vi "PH_Sequencer.ProcEvents.vi"(0 "i ref in":refnum<vi>, 5 "error in (no error)":errorcluster) -> (14 "i ref out":refnum<vi>, 19 "error out":errorcluster)   [LabVIEW 2014, in "PH_Sequencer.lvlib"]
doc: "This method is used to define the events the object will listen to. Add your own events here."
uses:
  PH_Sequencer.lvlib
  CS_Core/BaseProcess/BaseProcess.event definition.ctl
  CS_Core/CAEObj/CAEObj.event definition.ctl
  CS_Core/BaseProcess/BaseProcess.descriptor string definition.ctl
  PH_Basics/PH_PowerUnit_BaseClass/PH_PowerUnit_BaseClass.PP PU Tags.ctl
  PH_Basics/PH_PP_Common/PH_PP_Common.PUs.ctl
  PH_Devices/PH_Beckhoff_PP_PU/PH_Beckhoff_PP_PU.HV Meas Tags.ctl
  CS_Core/BaseProcess/BaseProcess.lvlib
  CS_Core/CAEObj/CAEObj.lvlib
  PH_Basics/PH_Common/PH_Common.lvlib
  PH_Devices/PH_Beckhoff_PP_PU/PH_Beckhoff_PP_PU.lvlib
  PH_Basics/PH_PowerUnit_BaseClass/PH_PowerUnit_BaseClass.lvlib
  PH_Basics/PH_PP_Common/PH_PP_Common.lvlib
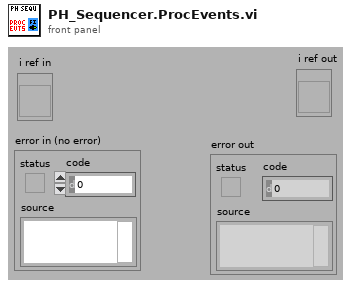
[diagram p1: front panel]
types:
  T1 = typedef "PH_PP_Common.lvlib/PH_PP_Common.PUs.ctl" = enum16{"no Info", "PA-19mm-1", "PA-19mm-2", "PA-45mm-PILC", "PA-45mm-MAIN", "MA-PU-1", "MA-PU-2", "MA-PU-3", "MA-PU-4", "MA-PU-5", "MA-PU-6", "MA-FR", "MA-PILC", "PA-45mm-DP"}
  T2 = typedef "PH_PowerUnit_BaseClass.lvlib/PH_PowerUnit_BaseClass.PP PU Tags.ctl" = enum16{"Waiting-Time", "PU-in-Use"}
  T3 = typedef "BaseProcess.lvlib/BaseProcess.event definition.ctl" = cluster{"CAEEvtDef":T4, "Data Descriptor":T5}
  T4 = typedef "CAEObj.lvlib/CAEObj.event definition.ctl" = cluster{"URL":string, "enable":bool, "ignoreResID":bool}
  T5 = typedef "BaseProcess.lvlib/BaseProcess.descriptor string definition.ctl" = string
  T6 = typedef "PH_Beckhoff_PP_PU.lvlib/PH_Beckhoff_PP_PU.HV Meas Tags.ctl" = enum16{"voltage-raw", "voltage"}
  T7 = typedef "PH_Sequencer.lvlib/PH_Sequencer.i attribute.ctl" = cluster{"GUI Refs":cluster{"Main Off":refnum<vi>, "Fire":refnum<vi>, "Status":refnum<vi>, "Ready":refnum<vi>, "Waiting Time":refnum<vi>, "Timeout":refnum<vi>, "PPMA Ready":refnum<vi>, "Sequencer SM State":refnum<vi>, "PPPA Ready":refnum<vi>, "Calorimeter":refnum<vi>, "Beamline Ready":refnum<vi>, "Clear Beamline":refnum<vi>, "Linkage PPMA Rods":refnum<vi>, "Linkage Current PA":refnum<vi>, "Linkage Current MA":refnum<vi>, "Timing Ready":refnum<vi>, "State Timing":refnum<vi>, "Force Timing":refnum<vi>, "PSDB Shot Comment":refnum<vi>, "State PA Backreflection":refnum<vi>, "Beamline Z6 Ready":refnum<vi>, "Clear Z6 Beamline":refnum<vi>, "Sequence length":refnum<vi>, "Timing Mode":refnum<vi>, "Slow Trigger Settings":refnum<vi>, "Experiment Description":refnum<vi>, "State PSDB":refnum<vi>, "PSDB Ready":refnum<vi>, "Set PSDB Settings":refnum<vi>, "Get PSDB Info":refnum<vi>, "Take Snapshot":refnum<vi>, "Shottype":refnum<vi>, "Experiment":refnum<vi>, "Phase Frontends":refnum<vi>, "PP 45mm PILC in use":refnum<vi>}, "Status Info":cluster{"Machine Status":T8, "WaitingTime":i32, "Timeout":bool}, "Readyness":cluster{"Ready to shot":bool, "PPMA Ready":bool, "PPPA Ready":bool, "BL Ready":bool, "Timing Ready":bool, "BL Z6 Ready":bool, "PSDBReady":bool}, "Instancenames":cluster{"PPMA Rods":string, "PP Current Meas":string, "PH Beamline Chief":string, "PA Backrefl Meas":string, "Z6 Beamline Chief":string}, "Data to read":bool, "Calorimeter":cluster{"Instancename":string, "On":bool, "linked":bool}, "Linkage":cluster{"PPMA Rods":bool, "PP Current Meas":bool, "PHELIX Beamline Chief":bool, "PA Backrefl Meas":bool, "Z6 Beamline Chief":bool}, "Timing":cluster{"Instance":string, "linked":bool, "Status":T8, "Timing Mode":T9, "Slow Trigger Settings":T10, "Info available":cluster{"ext SlowTrigger":bool, "T2":bool, "Mode":bool, "Delay Slow Trigger":bool, "Phase FEs":bool}, "FE Phase":T11}, "Service ID R2S":i32, "PSDB":cluster{"Controller Instance":string, "Controller Status":T8, "Controller linked":bool, "Settings acknowledged":bool, "Current Experiment ID":i16, "Current Shot Type":i16, "Current Comment":string, "Remember Settings":bool, "Write 2 early":bool}, "PSDB Data":cluster{"Main Off?":bool, "Sequence Length":dbl, "Sequence startet":timestamp}, "6P 4Q Positions":cluster{"Instancename":string, "linked":bool, "Position":T12}[], "PUs":T13[]}
  T8 = typedef "PH_StatusHandler.lvlib/PH_StatusHandler.Status.ctl" = i16
  T9 = typedef "PH_Timing.lvlib/PH_Timing.Timing Mode.ctl" = cluster{"T2":i16, "Modeselector":enum32{"10 Hz", "0.5 Hz", "Shot"}}
  T10 = typedef "PH_Timing.lvlib/PH_Timing.Slow Trigger Settings.ctl" = cluster{"Delay":dbl, "externally triggered?":bool}
  T11 = typedef "PH_Timing.lvlib/PH_Timing.Phase FEs.ctl" = cluster{"Phase":dbl}
  T12 = typedef "PH_4_Pos_Selector.lvlib/PH_4_Pos_Selector.Position Selector.ctl" = u16
  T13 = typedef "PH_Sequencer.lvlib/PH_Sequencer.Head.ctl" = cluster{"PowerUnit":T1, "GUI Ref":refnum<vi>, "Information":T14, "linked?":bool, "GUI Ref Current Voltage":refnum<vi>}
  T14 = typedef "PH_Sequencer.lvlib/PH_Sequencer.PU Information.ctl" = cluster{"State":T8, "Waiting Time [s]":dbl, "PU State SM":T15, "PU Timeout SM":T15}
  T15 = typedef "PH_PowerUnit_BaseClass.lvlib/PH_PowerUnit_BaseClass.SM States.ctl" = enum16{".", "Stand by", "Switch PU on", "Configure", "Set Default Voltage", "Set STANDBY", "Set READY", "Wait for Shot Cmd", "Open Dump Rods", "Open Ross Relais", "Close Ross Relais", "Switch PSU on", "Switch PSU off", "Charge", "Switch GD Channel on", "Close Dump Rods", "Rods-TO", "RR-TO", "PSU-TO", "Trigger-TO"}
  T16 = cluster{"Instancename":string, "linked":bool, "Position":T12}[]
  T17 = typedef "PH_Common.lvlib/PH_DIM.Event Declarer.ctl" = cluster{"Service Name":string, "Selector":string}
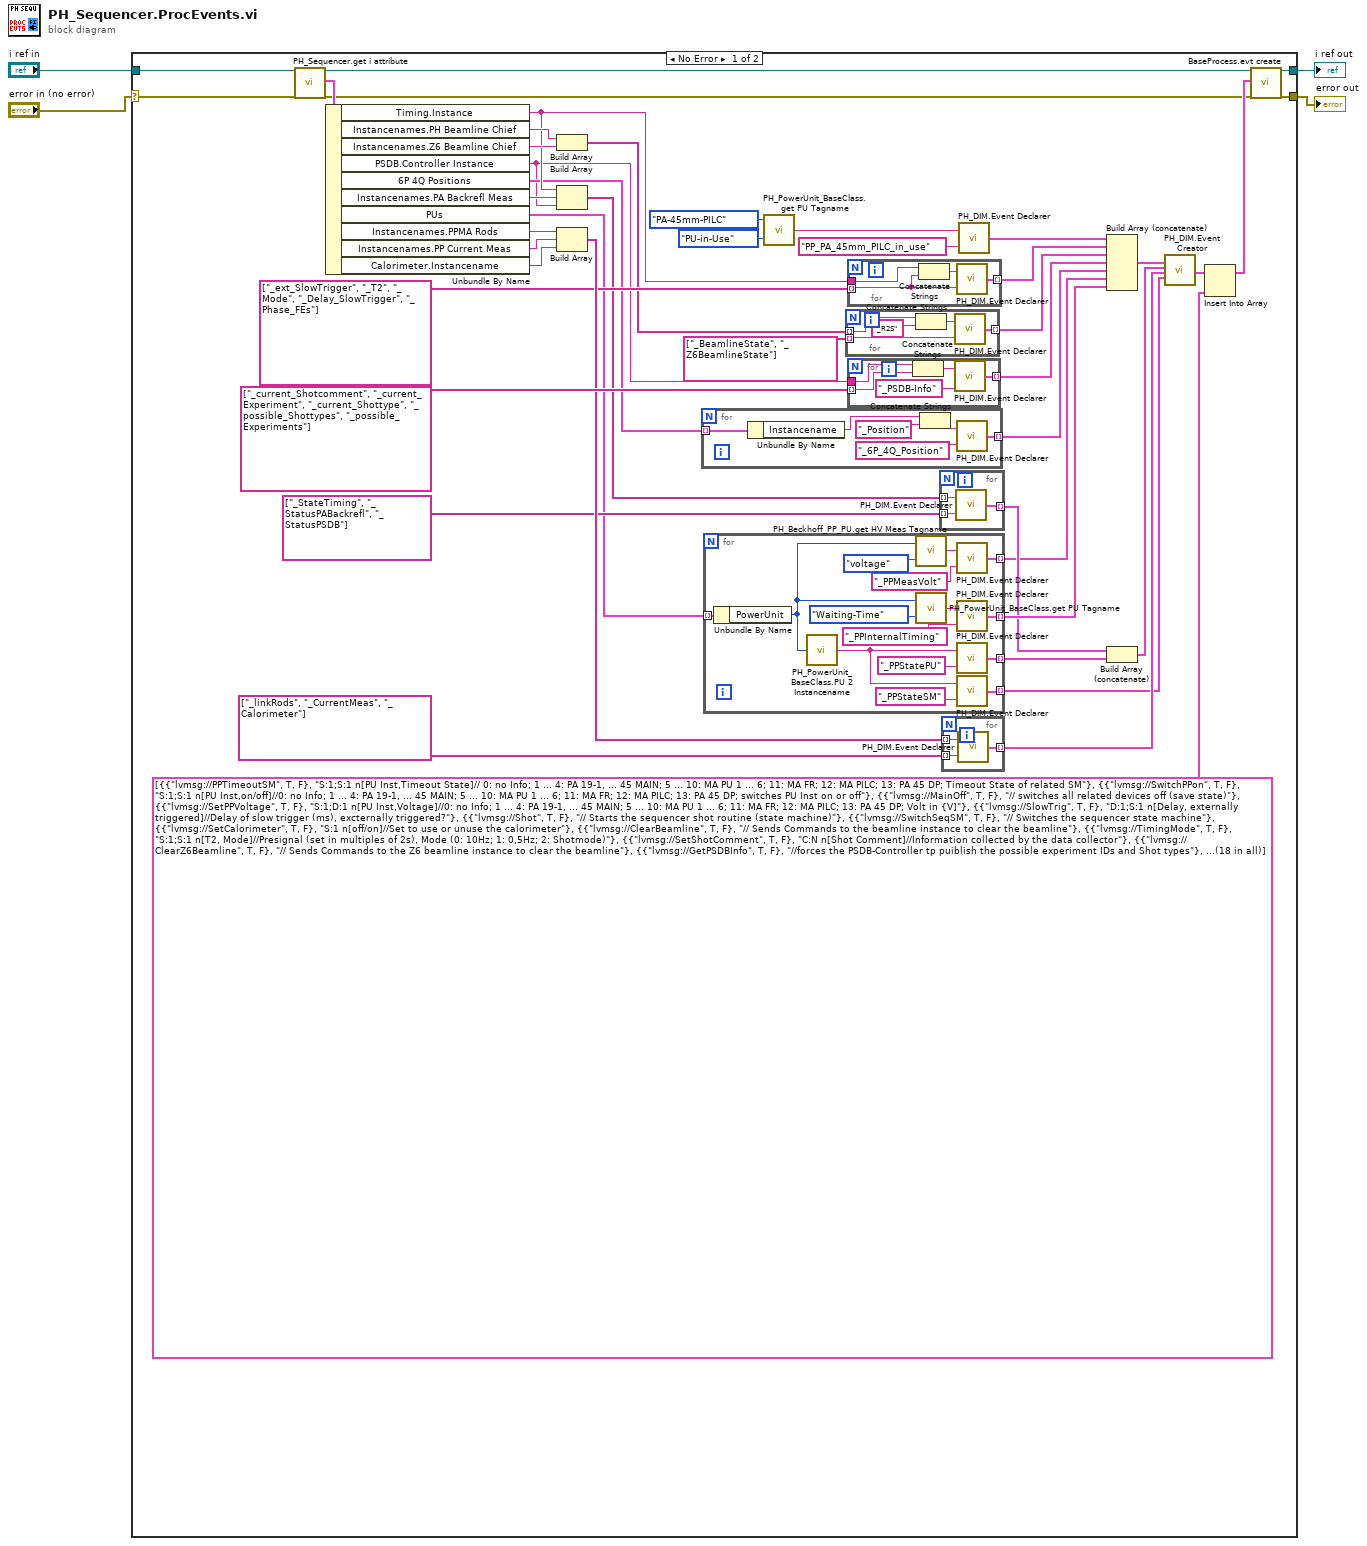
[diagram p0: block diagram]
diagram:
  n1 = case shown="No Error" "error in (no error)" {
    selector: "error in (no error)" -> [w44 w91]
    tunnel: "i ref in" -> [w47 w92]
    tunnel: [w46 w92] -> w3
    tunnel: [w45 w91] -> w2
    frame No Error {
      n2 = call "PH_Sequencer.get i attribute.vi"("i ref in"=w47, "error in (no error)"=w44) -> ("i ref out"=w49:refnum<vi>, "i attribute"=w32:T7, "error out"=w6:errorcluster)  [unwired: 15 in]
      n3 = Unbundle By Name(w32) -> ("Timing.Instance"=w21:string, "Instancenames.PH Beamline Chief"=w29:string, "Instancenames.Z6 Beamline Chief"=w28:string, "PSDB.Controller Instance"=w14:string, "6P 4Q Positions"=w18:T16, "Instancenames.PA Backrefl Meas"=w26:string, "PUs"=w16:T13[], "Instancenames.PPMA Rods"=w25:string, "Instancenames.PP Current Meas"=w24:string, "Calorimeter.Instancename"=w23:string)
      n4 = Build Array(w29, w28) -> (w13:string[])
      n5 = Build Array(w21, w26, w14) -> (w22:string[])
      n6 = Build Array(w25, w24, w23) -> (w38:string[])
      n7 = for {
        tunnel: [w53] -> w17 mode=indexing
        tunnel: w18 -> [w51] mode=indexing
        n8 = Unbundle By Name(w51) -> ("Instancename"=w50:string)
        n9 = Concatenate Strings(w50, "_Position" ("string")) -> (w55:string)
        n10 = call "PH_DIM.Event Declarer.vi"("Selector"="_6P_4Q_Position", "Service Name"=w55) -> ("declared DIM Event"=w53:T17)
      }
      n11 = for {
        tunnel: [w89] -> w39 mode=indexing
        tunnel: [w88] -> w34 mode=indexing
        tunnel: w16 -> [w86] mode=indexing
        tunnel: [w84] -> w9 mode=indexing
        tunnel: [w77] -> w8 mode=indexing
        n12 = Unbundle By Name(w86) -> ("PowerUnit"=w78:T1)
        n13 = call "PH_PowerUnit_BaseClass.PU 2 Instancename.vi"("PU"=w78) -> ("Instance Name"=w85:string)
        n14 = call "PH_Beckhoff_PP_PU.get HV Meas Tagname.vi"("HV Meas Tag"=PH_Beckhoff_PP_PU.HV_Meas_Tags."voltage", "PU"=w78) -> ("HV Meas Tagname"=w80:string)
        n15 = call "PH_PowerUnit_BaseClass.get PU Tagname.vi"("PU Tag"=PH_PowerUnit_BaseClass.PP_PU_Tags."Waiting-Time", "PU"=w78) -> ("PU Tagname"=w82:string)
        n16 = call "PH_DIM.Event Declarer.vi"("Selector"="_PPMeasVolt" ("URL"), "Service Name"=w80) -> ("declared DIM Event"=w77:T17)
        n17 = call "PH_DIM.Event Declarer.vi"("Selector"="_PPInternalTiming" ("URL"), "Service Name"=w82) -> ("declared DIM Event"=w89:T17)
        n18 = call "PH_DIM.Event Declarer.vi"("Selector"="_PPStatePU" ("URL"), "Service Name"=w85) -> ("declared DIM Event"=w88:T17)
        n19 = call "PH_DIM.Event Declarer.vi"("Selector"="_PPStateSM" ("URL"), "Service Name"=w85) -> ("declared DIM Event"=w84:T17)
      }
      n20 = call "PH_PowerUnit_BaseClass.get PU Tagname.vi"("PU Tag"=PH_PowerUnit_BaseClass.PP_PU_Tags."PU-in-Use", "PU"=PH_PP_Common.PUs."PA-45mm-PILC") -> ("PU Tagname"=w11:string)
      n21 = for {
        tunnel: [w75] -> w40 mode=indexing
        tunnel: w13 -> [w73] mode=indexing
        tunnel: string[] ["_BeamlineState", "_Z6BeamlineState"] -> [w74] mode=indexing
        n22 = Concatenate Strings(w73, "_R2S" ("string")) -> (w72:string)
        n23 = call "PH_DIM.Event Declarer.vi"("Selector"=w74, "Service Name"=w72) -> ("declared DIM Event"=w75:T17)
      }
      n24 = for {
        tunnel: [w59] -> w27 mode=indexing
        tunnel: w21 -> [w57]
        tunnel: string[] ["_ext_SlowTrigger", "_T2", "_Mode", "_Delay_SlowTrigger", "_Phase_FEs"] -> [w56] mode=indexing
        n25 = Concatenate Strings(w57, w56) -> (w58:string)
        n26 = call "PH_DIM.Event Declarer.vi"("Selector"=w56, "Service Name"=w58) -> ("declared DIM Event"=w59:T17)
      }
      n27 = for {
        tunnel: w14 -> [w64]
        tunnel: string[] ["_current_Shotcomment", "_current_Experiment", "_current_Shottype", "_possible_Shottypes", "_possible_Experiments"] -> [w63] mode=indexing
        tunnel: [w60] -> w41 mode=indexing
        n28 = Concatenate Strings(w64, w63) -> (w62:string)
        n29 = call "PH_DIM.Event Declarer.vi"("Selector"="_PSDB-Info" ("URL"), "Service Name"=w62) -> ("declared DIM Event"=w60:T17)
      }
      n30 = for {
        tunnel: [w65] -> w35 mode=indexing
        tunnel: w22 -> [w67] mode=indexing
        tunnel: string[] ["_StateTiming", "_StatusPABackrefl", "_StatusPSDB"] -> [w66] mode=indexing
        n31 = call "PH_DIM.Event Declarer.vi"("Selector"=w66, "Service Name"=w67) -> ("declared DIM Event"=w65:T17)
      }
      n32 = for {
        tunnel: [w68] -> w15 mode=indexing
        tunnel: w38 -> [w69] mode=indexing
        tunnel: string[] ["_linkRods", "_CurrentMeas", "_Calorimeter"] -> [w70] mode=indexing
        n33 = call "PH_DIM.Event Declarer.vi"("Selector"=w70, "Service Name"=w69) -> ("declared DIM Event"=w68:T17)
      }
      n34 = call "PH_DIM.Event Declarer.vi"("Selector"="PP_PA_45mm_PILC_in_use", "Service Name"=w11) -> ("declared DIM Event"=w7:T17)
      n35 = Build Array (concatenate)(w7, w27, w40, w41, w17, w8, w39) -> (w42:T17[])
      n36 = Build Array (concatenate)(w35, w34) -> (w36:T17[])
      n37 = call "PH_DIM.Event Creator.vi"("Trendmessage Services"=w42, "Status Services"=w36, "condition Services"=w15, "SM State Services"=w9) -> ("DIM Service Events"=w20:T3[])  [unwired: 15 in]
      n38 = Insert Into Array(array=w20, new element=T3[] [{"CAEEvtDef"={"URL"="lvmsg://PPTimeoutSM", "enable"=TRUE, "ignoreResID"=FALSE}, "Data Descriptor"="S:1;S:1 n[PU Inst,Timeout State]// 0: no Info; 1 ... 4: PA 19-1, ... 45 MAIN; 5 ... 10: MA PU 1 ... 6; 11: MA FR; 12: MA PILC; 13: PA 45 DP; Timeout State of related SM"}, {"CAEEvtDef"={"URL"="lvmsg://SwitchPPon", "enable"=TRUE, "ignoreResID"=FALSE}, "Data Descriptor"="S:1;S:1 n[PU Inst,on/off]//0: no Info; 1 ... 4: PA 19-1, ... 45 MAIN; 5 ... 10: MA PU 1 ... 6; 11: MA FR; 12: MA PILC; 13: PA 45 DP; switches PU Inst on or off"}, {"CAEEvtDef"={"URL"="lvmsg://MainOff", "enable"=TRUE, "ignoreResID"=FALSE}, "Data Descriptor"="// switches all related devices off (save state)"}, {"CAEEvtDef"={"URL"="lvmsg://SetPPVoltage", "enable"=TRUE, "ignoreResID"=FALSE}, "Data Descriptor"="S:1;D:1 n[PU Inst,Voltage]//0: no Info; 1 ... 4: PA 19-1, ... 45 MAIN; 5 ... 10: MA PU 1 ... 6; 11: MA FR; 12: MA PILC; 13: PA 45 DP; Volt in {V]"}, {"CAEEvtDef"={"URL"="lvmsg://SlowTrig", "enable"=TRUE, "ignoreResID"=FALSE}, "Data Descriptor"="D:1;S:1 n[Delay, externally triggered]//Delay of slow trigger (ms), excternally triggered?"}, {"CAEEvtDef"={"URL"="lvmsg://Shot", "enable"=TRUE, "ignoreResID"=FALSE}, "Data Descriptor"="// Starts the sequencer shot routine (state machine)"}, {"CAEEvtDef"={"URL"="lvmsg://SwitchSeqSM", "enable"=TRUE, "ignoreResID"=FALSE}, "Data Descriptor"="// Switches the sequencer state machine"}, {"CAEEvtDef"={"URL"="lvmsg://SetCalorimeter", "enable"=TRUE, "ignoreResID"=FALSE}, "Data Descriptor"="S:1 n[off/on]//Set to use or unuse the calorimeter"}, {"CAEEvtDef"={"URL"="lvmsg://ClearBeamline", "enable"=TRUE, "ignoreResID"=FALSE}, "Data Descriptor"="// Sends Commands to the beamline instance to clear the beamline"}, {"CAEEvtDef"={"URL"="lvmsg://TimingMode", "enable"=TRUE, "ignoreResID"=FALSE}, "Data Descriptor"="S:1;S:1 n[T2, Mode]//Presignal (set in multiples of 2s), Mode (0: 10Hz; 1: 0,5Hz; 2: Shotmode)"}, {"CAEEvtDef"={"URL"="lvmsg://SetShotComment", "enable"=TRUE, "ignoreResID"=FALSE}, "Data Descriptor"="C:N n[Shot Comment]//Information collected by the data collector"}, {"CAEEvtDef"={"URL"="lvmsg://ClearZ6Beamline", "enable"=TRUE, "ignoreResID"=FALSE}, "Data Descriptor"="// Sends Commands to the Z6 beamline instance to clear the beamline"}, {"CAEEvtDef"={"URL"="lvmsg://GetPSDBInfo", "enable"=TRUE, "ignoreResID"=FALSE}, "Data Descriptor"="//forces the PSDB-Controller tp puiblish the possible experiment IDs and Shot types"}, {"CAEEvtDef"={"URL"="lvmsg://SetExpID", "enable"=TRUE, "ignoreResID"=FALSE}, "Data Descriptor"="S:1 n[Experiment ID]//sends the wanted Experiment ID to the PSDB-Controller"}, {"CAEEvtDef"={"URL"="lvmsg://SetShotType", "enable"=TRUE, "ignoreResID"=FALSE}, "Data Descriptor"="S:1 n[Shot Type]//sends the wanted Shot Type to the PSDB-Controller"}, {"CAEEvtDef"={"URL"="lvmsg://SetPSDBSettings", "enable"=TRUE, "ignoreResID"=FALSE}, "Data Descriptor"="// confirms by setting own attributes that PSDB-Settings are checked"}, {"CAEEvtDef"={"URL"="lvmsg://GetPSDBSnapshot", "enable"=TRUE, "ignoreResID"=FALSE}, "Data Descriptor"="// requests a PSDB Snapshot"}, {"CAEEvtDef"={"URL"="lvmsg://PhaseFEs", "enable"=TRUE, "ignoreResID"=FALSE}, "Data Descriptor"="D:1 n[Phase]//Sets the phase between the frontends in seconds"}] ("new events")) -> (w48:T3[])  [unwired: 1 in]
      n39 = call "BaseProcess.evt create.vi"("i ref in"=w49, "newEvents"=w48, "error in (no error)"=w6) -> ("i ref out"=w46:refnum<vi>, "error out"=w45:errorcluster)  [unwired: 13 in, 2 out]
    }
    frame Error {
    }
  }
  "i ref out" <- w3
  "error out" <- w2
